vi "Bone_Init.vi"(3 "error in":errorcluster, 4 "Task":enum16{"Init", "Close"}(ring)) -> (0 "error out":errorcluster, 1 "String":string)   [LabVIEW 2012]
uses:
  <userlib>/BotSpeak/VIs/Direct/BotSpeak_Control.ctl
panel:
  in  "Connection In":T1
  out "Connection Out":T1
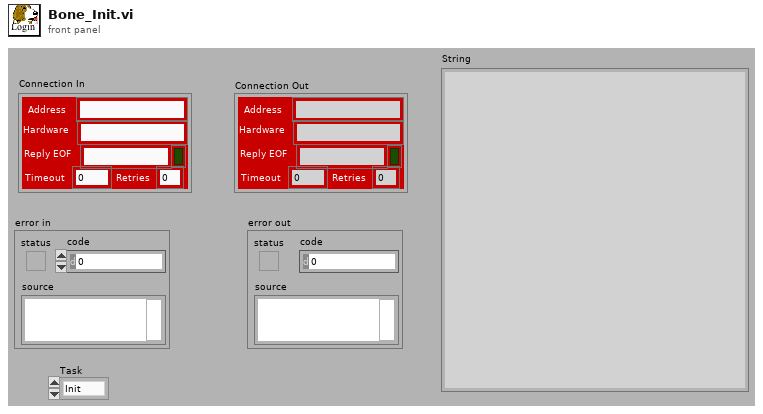
[diagram p1: front panel]
types:
  T1 = typedef "BotSpeak_Control.ctl" = cluster{"Address":string, "Reply EOF":string, "Hardware":string, "Retries":i8, "Timeout":i32, "Open?":bool}
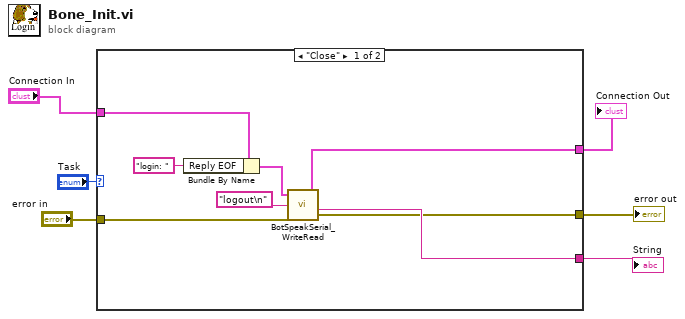
[diagram p0: block diagram]
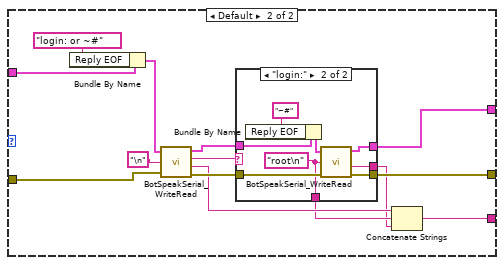
[diagram p2: hidden frame]
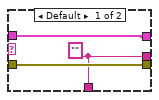
[diagram p3: hidden frame]
diagram:
  n1 = case shown="\"Close\"" "Task" {
    tunnel: [w13 w28] -> w6
    tunnel: [w11 w26] -> w2
    tunnel: "Connection In" -> [w10 w23]
    tunnel: [w14 w18] -> w5
    tunnel: "error in" -> [w12 w16]
    frame "Close" {
      n2 = Bundle By Name(cluster=w10, "Reply EOF"="login: " ("Bot Settings.Reply EOF")) -> (w7:T1)
      n3 = call <userlib>:"BotSpeakSerial_WriteRead.vi"("error In"=w12, "To Write"="logout\n" ("String To Send"), "Bot Settings in"=w7) -> ("error out"=w13:errorcluster, "Reply"=w14:string, "Bot Settings out"=w11:T1)  [unwired: 1 out]
    }
    frame Default {
      n4 = Bundle By Name(cluster=w23, "Reply EOF"="login: or ~#" ("Status String")) -> (w15:T1)
      n5 = call <userlib>:"BotSpeakSerial_WriteRead.vi"("error In"=w16, "To Write"="\n" ("Status String"), "Bot Settings in"=w15) -> ("error out"=w27:errorcluster, "Reply"=w21:string, "Reply EOF"=w17:string, "Bot Settings out"=w25:T1)
      n6 = case shown="\"login:\"" w17 {
        tunnel: [w30 w39] -> w28
        tunnel: w27 -> [w30 w38]
        tunnel: [w31 w37] -> w26
        tunnel: w25 -> [w31 w34]
        tunnel: [w29 w33] -> w20
        tunnel: [w29 w32] -> w19
        frame Default {
          w29 = "" ("Status String")
        }
        frame "login:" {
          w33 = "root\n" ("Status String")
          n7 = Bundle By Name(cluster=w34, "Reply EOF"="~#" ("Status String")) -> (w36:T1)
          n8 = call <userlib>:"BotSpeakSerial_WriteRead.vi"("error In"=w38, "To Write"=w33, "Bot Settings in"=w36) -> ("error out"=w39:errorcluster, "Reply"=w32:string, "Bot Settings out"=w37:T1)  [unwired: 1 out]
        }
      }
      n9 = Concatenate Strings(w21, w20, w19) -> (w18:string)
    }
  }
  "error out" <- w6
  "String" <- w5
  "Connection Out" <- w2
